vi "mod_Create Profile.vi"(9 "interpolation":T1(ring)=enum."linear dB", 10 "dt":dbl=1.0 format="%.2p", 11 "profile definition":cluster{"time":dbl, "power (dB)":dbl}[](array[cluster]) {"power (dB)" format="%.2f"; "time" format="%.2f"}) -> (3 "profile":dbl[](array[numeric]) format="%.2f")   [LabVIEW 2020, in "niDMT.lvlib"]
uses:
  <vilib>/addons/Modulation/niDMT.lvlib
  <vilib>/ptbypt/NI_PtbyPt.lvlib
panel:
  out "Waveform Graph":dbl[](graph)
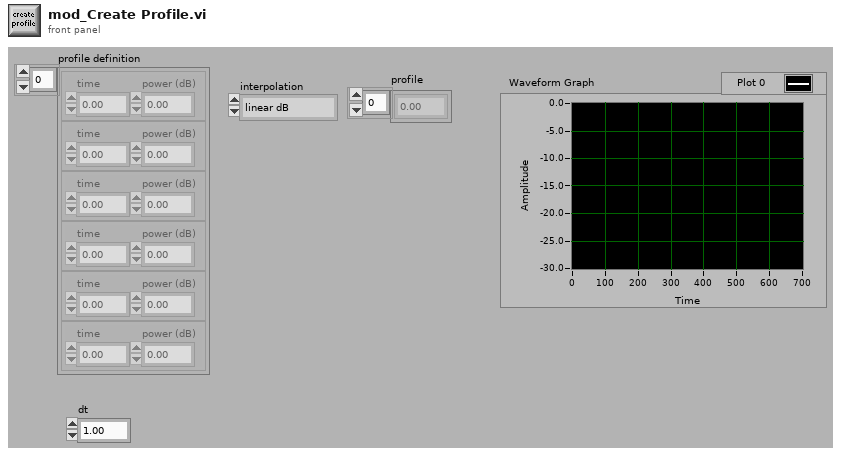
[diagram p1: front panel]
types:
  T1 = enum16{"linear power", "linear voltage", "linear dB"}
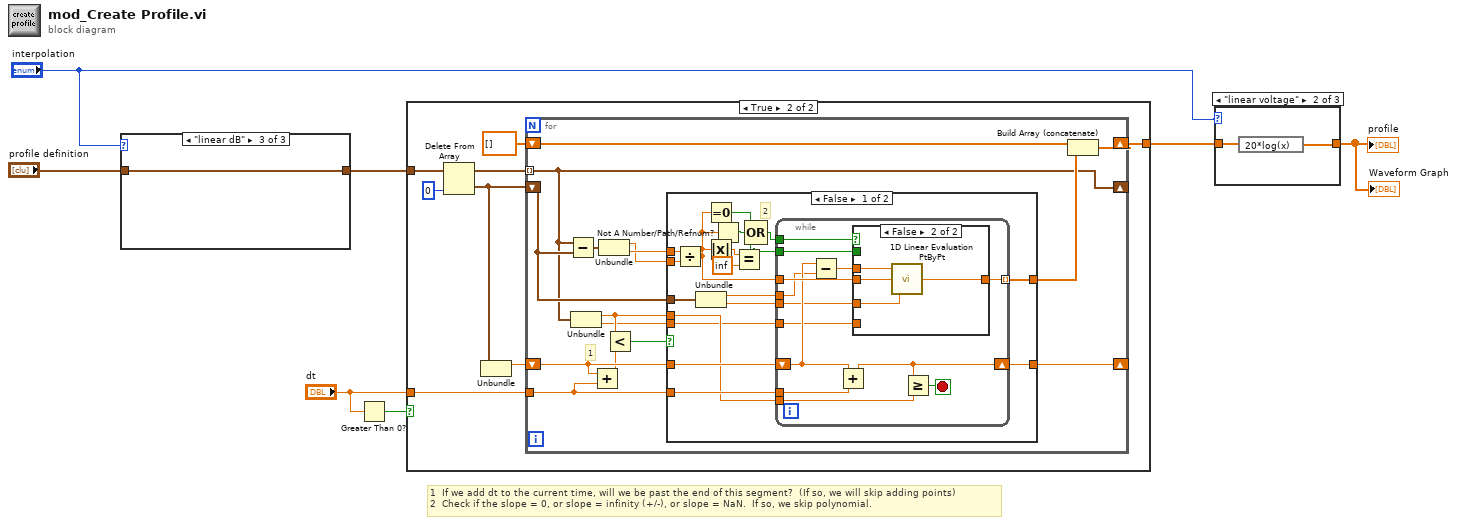
[diagram p0: block diagram]
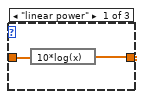
[diagram p2: hidden frame]
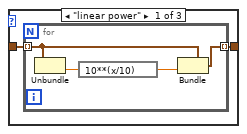
[diagram p4: hidden frame]
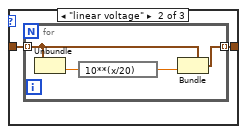
[diagram p5: hidden frame]
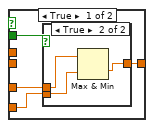
[diagram p7: hidden frame]
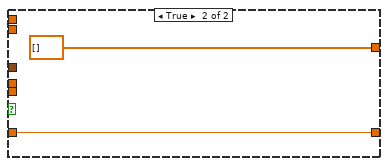
[diagram p9: hidden frame]
diagram:
  # "1  If we add dt to the current time, will we be past the end of this segment?  (If so, we will skip adding points)\n2  Check if the slope = 0, or slope = infinity (+/-), or slope = NaN.  If so, we skip polynomial."
  n1 = case shown="\"linear dB\"" "interpolation" {
    tunnel: "profile definition" -> [w9 w15 w20]
    tunnel: [w8 w14 w20] -> w4
    frame "linear power" {
      n2 = for {
        tunnel: w9 -> [w11] mode=indexing
        tunnel: [w10] -> w8 mode=indexing
        n3 = Unbundle(w11) -> ("power (dB)"=w13:dbl)  [unwired: 1 out]
        n4 = expression code="10**(x/10)"(w13) -> (w12:dbl)
        n5 = Bundle(cluster=w11, "power (dB)"=w12) -> (w10:cluster{"time":dbl, "power (dB)":dbl})  [unwired: 1 out]
      }
    }
    frame "linear voltage" {
      n6 = for {
        tunnel: w15 -> [w17] mode=indexing
        tunnel: [w16] -> w14 mode=indexing
        n7 = Unbundle(w17) -> ("power (dB)"=w19:dbl)  [unwired: 1 out]
        n8 = expression code="10**(x/20)"(w19) -> (w18:dbl)
        n9 = Bundle(cluster=w17, "power (dB)"=w18) -> (w16:cluster{"time":dbl, "power (dB)":dbl})  [unwired: 1 out]
      }
    }
    frame "linear dB" {
    }
  }
  n10 = Greater Than 0?(x="dt") -> (x > 0?=w6:bool)
  n11 = case shown="True" w6 {
    tunnel: "dt" -> [_ w28]
    tunnel: w4 -> [_ w25]
    tunnel: [_ w22] -> w2
    frame False {
    }
    frame True {
      n12 = Delete From Array(array=w25, index=0) -> (deleted portion=w27:cluster{"time":dbl, "power (dB)":dbl}, array with subset deleted=w23:cluster{"time":dbl, "power (dB)":dbl}[])  [unwired: 1 in]
      n13 = Unbundle(w27) -> ("time"=w26:dbl)  [unwired: 1 out]
      n14 = for {
        tunnel: w28 -> [w34]
        shift-right: [w43] -> w22
        shift-left: dbl[] [] -> [w42]
        shift-right: [w32] -> _
        shift-left: w27 -> [w36]
        tunnel: w23 -> [w32] mode=indexing
        shift-right: [w37] -> _
        shift-left: w26 -> [w35]
        # "1"
        n15 = Subtract(x=w32, y=w36) -> (x-y=w41:cluster{"time":dbl, "power (dB)":dbl})
        n16 = Unbundle(w32) -> ("time"=w31:dbl, "power (dB)"=w30:dbl)
        n17 = Add(x=w35, y=w34) -> (x+y=w33:dbl)
        n18 = Unbundle(w41) -> ("time"=w38:dbl, "power (dB)"=w39:dbl)
        n19 = Less?(x=w31, y=w33) -> (x < y?=w29:bool)
        n20 = case shown="False" w29 {
          tunnel: w34 -> [w61 _]
          tunnel: w35 -> [w60 w88]
          tunnel: [w59 dbl[] []] -> w40
          tunnel: w39 -> [w54 _]
          tunnel: w38 -> [w58 _]
          tunnel: [w57 w88] -> w37
          tunnel: w36 -> [w56 _]
          tunnel: w31 -> [w52 _]
          tunnel: w30 -> [w47 _]
          frame False {
            # "2"
            n21 = Divide(x=w54, y=w58) -> (x/y=w46:dbl)
            n22 = Unbundle(w56) -> ("time"=w53:dbl, "power (dB)"=w55:dbl)
            n23 = Equal To 0?(x=w46) -> (x = 0?=w51:bool)
            n24 = Absolute Value(x=w46) -> (abs(x)=w49:dbl)
            n25 = Not A Number/Path/Refnum?(number/path/refnum=w46) -> (NaN/Path/Refnum?=w45:bool)
            n26 = Equal?(x=w49, y=inf) -> (x = y?=w48:bool)
            n27 = Compound Arithmetic op=OR(w51, w45, w48) -> (w50:bool)
            n28 = while {
              shift-right: [w67] -> w57
              shift-left: w60 -> [w71]
              tunnel: w61 -> [w74]
              tunnel: [w73] -> w59 mode=indexing
              tunnel: w46 -> [w72]
              tunnel: w55 -> [w69]
              tunnel: w53 -> [w68]
              tunnel: w52 -> [w66]
              tunnel: w50 -> [w64]
              tunnel: w48 -> [w63]
              tunnel: w47 -> [w62]
              stop <- w65 stop-if-true
              n29 = Subtract(x=w71, y=w68) -> (x-y=w70:dbl)
              n30 = Add(x=w71, y=w74) -> (x+y=w67:dbl)
              n31 = case shown="False" w64 {
                tunnel: w70 -> [_ w86]
                tunnel: [w75 w83] -> w73
                tunnel: w72 -> [_ w85]
                tunnel: w69 -> [w76 w84]
                tunnel: w63 -> [w78 _]
                tunnel: w62 -> [w77 _]
                frame True {
                  n32 = case shown="True" w78 {
                    tunnel: w77 -> [_ w81]
                    tunnel: w76 -> [w79 w82]
                    tunnel: [w79 w80] -> w75
                    frame False {
                    }
                    frame True {
                      n33 = Max & Min(x=w82, y=w81) -> (min(x,y)=w80:dbl)  [unwired: 1 out]
                    }
                  }
                }
                frame False {
                  n34 = call <vilib>:"1D Linear Evaluation PtByPt.vi"("offset"=w84, "scale"=w85, "x"=w86) -> ("y[i]=x[i]*a+b"=w83:dbl)
                }
              }
              n35 = Greater Or Equal?(x=w67, y=w66) -> (x >= y?=w65:bool)
            }
          }
          frame True {
          }
        }
        n36 = Build Array (concatenate)(w42, w40) -> (w43:dbl[])
      }
    }
  }
  n37 = case shown="\"linear voltage\"" "interpolation" {
    tunnel: w2 -> [w90 w92 w93]
    tunnel: [w89 w91 w93] -> w1
    frame "linear power" {
      n38 = expression code="10*log(x)"(w90) -> (w89:dbl[])
    }
    frame "linear voltage" {
      n39 = expression code="20*log(x)"(w92) -> (w91:dbl[])
    }
    frame "linear dB" {
    }
  }
  "profile" <- w1
  "Waveform Graph" <- w1
